vi "GDSAPI_UpdateAttributes.vi"(8 "error in (no error)":errorcluster, 9 "DeleteAllPreviousAttributes(True)":bool=TRUE, 10 "Attributes(Name : Type)":string[](array[string]), 11 "OriginalClassPath(*.lvclass)":path) -> (0 "error out":errorcluster)   [LabVIEW 2020]
doc: "This VI updates the attributes of a class."
uses:
  <resource>/Framework/Providers/Open_GDS/ClassProviders/Provider_BaseClassInterface/ClassReader_class/ClassReader.lvclass
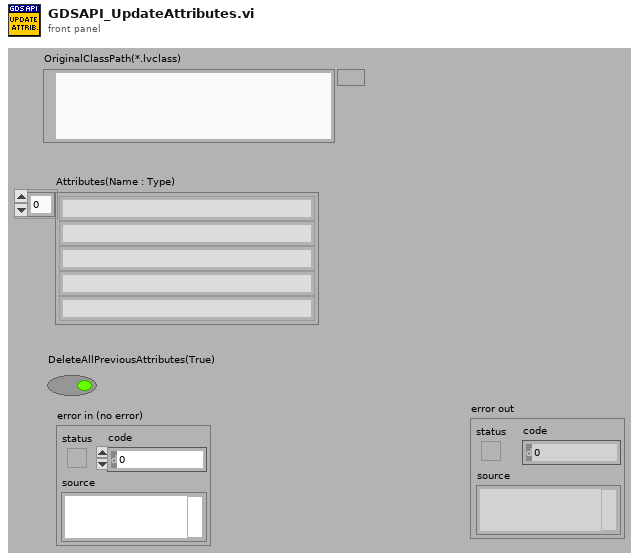
[diagram p1: front panel]
types:
  T1 = typedef "ReversedEngineering AttributeInfoType.ctl" = cluster{"name":string, "type":T2, "dimension":i32, "typeName":string, "typePath":path, "visibility":T3}
  T2 = typedef "CommonVIs_AttributeDataType.ctl" = enum16{"UINT8", "INT8", "UINT16", "INT16", "UINT32", "INT32", "UINT64", "INT64", "SGL", "DBL", "EXT", "CSG", "CDB", "CXT", "TimeStamp", "STRING", "PATH", "BOOL", "ENUM", "RefNum", "VIRefNum", "LabVIEW Class", "Cluster", "Variant", "TypeDef", "Waveform", "LabVIEW Object", "Other", "void"}
  T3 = typedef "UMLEditor_VisibilityType.ctl" = enum16{"Public", "Private", "Protected"}
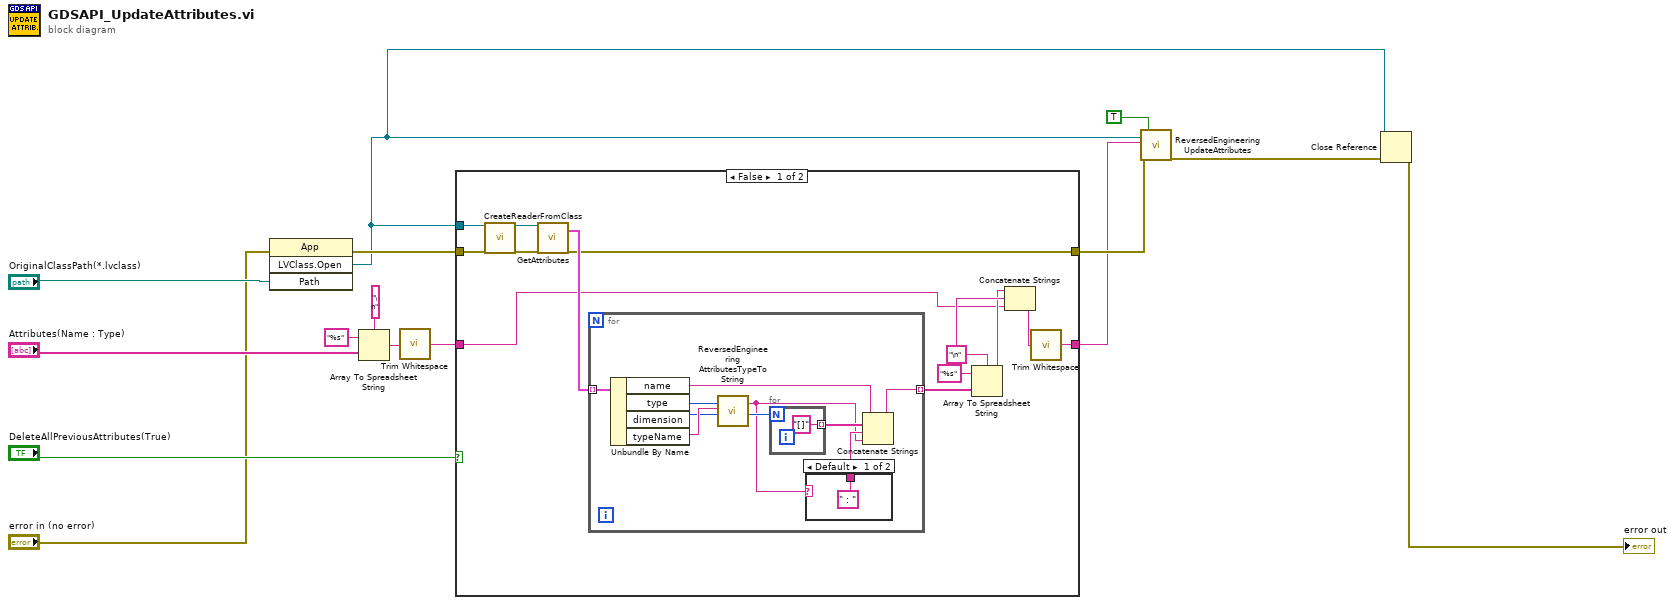
[diagram p0: block diagram]
diagram:
  n1 = invoke class="App" method="LVClass.Open"(error in="error in (no error)", "Path"="OriginalClassPath(*.lvclass)") -> (error out=w5:errorcluster, "LVClass.Open"=w3:refnum<vi>)  [unwired: 2 in, 2 out]
  n2 = Array To Spreadsheet String(delimiter (Tab)="\n", array="Attributes(Name : Type)", 3:"%s" ("format string")) -> (spreadsheet string=w8:string)
  n3 = call <vilib>:"Trim Whitespace.vi"("string"=w8) -> ("trimmed string"=w6:string)  [unwired: 1 in]
  n4 = case shown="False" "DeleteAllPreviousAttributes(True)" {
    tunnel: w6 -> [w16 w41]
    tunnel: [w19 w41] -> w2
    tunnel: w5 -> [w26 w40]
    tunnel: [w18 w40] -> w4
    tunnel: w3 -> [w25 _]
    frame False {
      w21 = "\n" ("delimiter (Tab)")
      n5 = call <resource>:"CreateReaderFromClass.vi"("ClassPath/LvClassRef"=w25, "error in"=w26) -> ("ClassReader"=w28:refnum<class "ClassReader.lvclass">, "error out"=w27:errorcluster)  [unwired: 14 in, 2 out]
      n6 = call-dynamic "GetAttributes.vi"("ClassReader in"=w28, "error in (no error)"=w27) -> ("ObjectAttributes"=w22:T1[], "error out"=w18:errorcluster)  [unwired: 12 in, 4 out]
      n7 = for {
        tunnel: w22 -> [w37] mode=indexing
        tunnel: [w30] -> w24 mode=indexing
        n8 = Unbundle By Name(w37) -> ("name"=w31:string, "type"=w36:T2, "dimension"=w34:i32, "typeName"=w35:string)
        n9 = call <resource>:"ReversedEngineering AttributesTypeToString.vi"("AttributeDataType"=w36, "name"=w35) -> ("string"=w29:string)  [unwired: 17 in]
        n10 = for {
          N: w34 -> [_]
          tunnel: ["[]"] -> w33 mode=indexing
        }
        n11 = case shown="Default" w29 {
          tunnel: [" : " _] -> w32
          frame Default {
          }
          frame "" {
          }
        }
        n12 = Concatenate Strings(w31, w33, w32, w29) -> (w30:string)
      }
      n13 = Array To Spreadsheet String(delimiter (Tab)=w21, array=w24, 3:"%s" ("format string")) -> (spreadsheet string=w17:string)
      n14 = Concatenate Strings(w17, w21, w16) -> (w20:string)
      n15 = call <vilib>:"Trim Whitespace.vi"("string"=w20) -> ("trimmed string"=w19:string)  [unwired: 1 in]
    }
    frame True {
    }
  }
  n16 = call <resource>:"ReversedEngineering UpdateAttributes.vi"("ClassPath/LvClassRef"=w3, "NewAttributes"=w2, "error in (no error)"=w4, "Don't Prompt (False)"=TRUE) -> ("error out"=w7:errorcluster)  [unwired: 13 in, 2 out]
  n17 = Close Reference(reference=w3, error in (no error)=w7) -> (error out=→"error out":errorcluster)
